vi "Rate scan.vi"(6 "T Ventana":u32 format="%x", 7 "Espera acceso USB":u32, 8 "error in 2":errorcluster, 9 "Valor buscado scalers (5000)":u16, 10 "Sumador":u8, 11 "ftHandle_in 2":u32) -> (0 "error out 2":errorcluster, 1 "DAC\nTH3,TH4,TH5":u16 format="%x", 2 "DAC\nTH0,TH1,TH2":u16 format="%x", 3 "ftHandle_out 2":u32, 5 "Scaler 1":u16)   [LabVIEW 2019]
uses:
  Origen Socket SERVO_PCB_BUENO_v5 (muchos asics)/Global_STOP.vi
panel:
  out "Scaler 2":u16
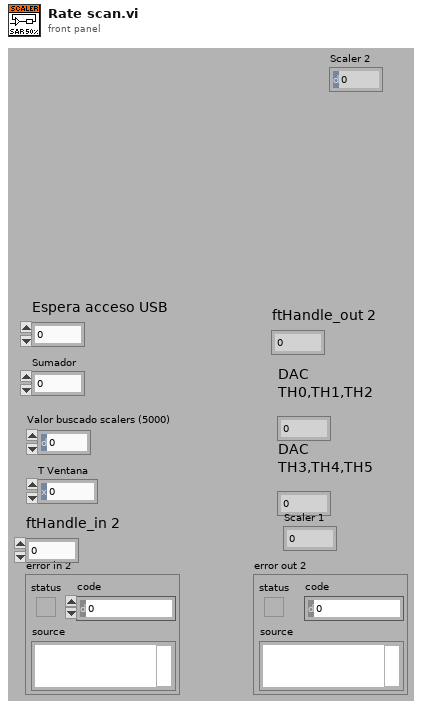
[diagram p1: front panel]
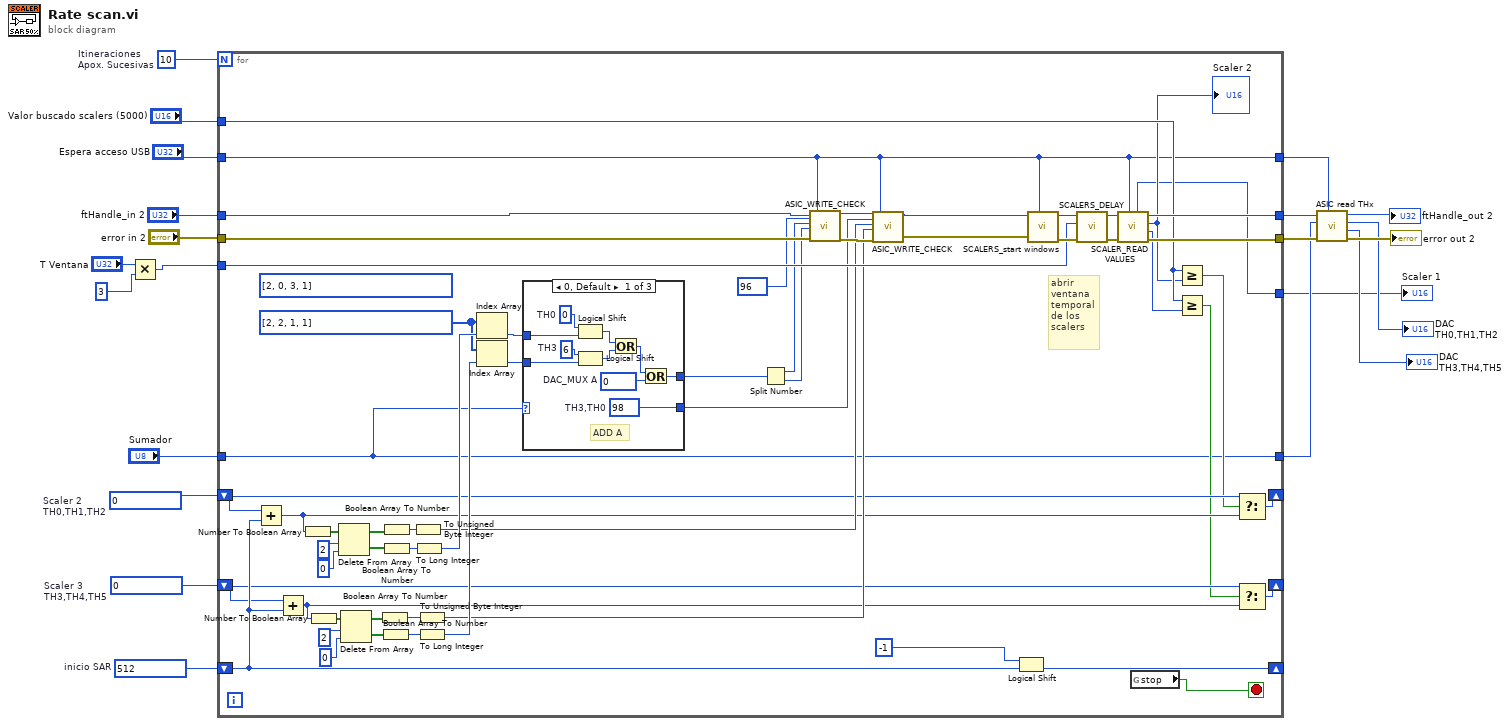
[diagram p0: block diagram]
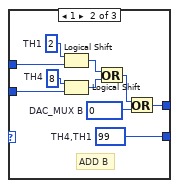
[diagram p2: hidden frame]
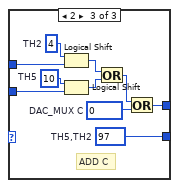
[diagram p3: hidden frame]
diagram:
  w14 = u16 0  # Scaler 3 TH3,TH4,TH5
  w15 = u16 0  # Scaler 2 TH0,TH1,TH2
  w16 = u16 512  # inicio SAR
  w18 = 10  # Itineraciones Apox. Sucesivas
  n1 = Multiply(x="T Ventana", y=u32 3) -> (x*y=w2:u32)
  n2 = for {
    N: w18 -> [_]
    tunnel: "Espera acceso USB" -> [w26]
    tunnel: w2 -> [w76]
    tunnel: "Valor buscado scalers (5000)" -> [w28]
    shift-right: [w72] -> _
    shift-left: w16 -> [w71]
    shift-right: [w33] -> _
    shift-left: w15 -> [w40]
    shift-right: [w32] -> _
    shift-left: w14 -> [w38]
    tunnel: "Sumador" -> [w30]
    tunnel: [w30] -> w9
    tunnel: [w26] -> w10
    tunnel: [w25] -> w4
    tunnel: "ftHandle_in 2" -> [w54]
    tunnel: [w35] -> w11
    tunnel: "error in 2" -> [w53]
    tunnel: [w34] -> w12
    stop <- w22 stop-if-true
    (unwired) u16[] [2, 0, 3, 1]
    w51 = u16[] [2, 2, 1, 1]
    # "abrir ventana temporal de los scalers"
    n3 = Add(x=w40, y=w71) -> (x+y=w39:u16)
    n4 = Add(x=w38, y=w71) -> (x+y=w37:u16)
    n5 = Number To Boolean Array(number=w39) -> (Boolean array=w70:bool[])
    n6 = Number To Boolean Array(number=w37) -> (Boolean array=w69:bool[])
    n7 = Delete From Array(array=w70, length=2, index=0) -> (deleted portion=w63:bool[], array with subset deleted=w68:bool[])
    n8 = Delete From Array(array=w69, length=2, index=0) -> (deleted portion=w61:bool[], array with subset deleted=w62:bool[])
    n9 = Boolean Array To Number(Boolean array=w62) -> (number=w59:u32)
    n10 = Boolean Array To Number(Boolean array=w61) -> (number=w57:u32)
    n11 = Boolean Array To Number(Boolean array=w68) -> (number=w60:u32)
    n12 = Boolean Array To Number(Boolean array=w63) -> (number=w58:u32)
    n13 = To Unsigned Byte Integer(number=w60) -> (unsigned 8bit integer=w42:u8)
    n14 = To Long Integer(number=w58) -> (32bit integer=w56:i32)
    n15 = To Unsigned Byte Integer(number=w59) -> (unsigned 8bit integer=w41:u8)
    n16 = To Long Integer(number=w57) -> (32bit integer=w55:i32)
    n17 = Index Array(array=w51, index=w56) -> (element=w50:u16)
    n18 = Index Array(array=w51, index=w55) -> (element=w49:u16)
    n19 = case shown="0, Default" w30 {
      tunnel: [w88 w98 w108] -> w43
      tunnel: w50 -> [w87 w97 w107]
      tunnel: w49 -> [w86 w96 w106]
      tunnel: [w80 w90 w100] -> w44
      frame 0, Default {
        w79 = u16 0  # DAC_MUX A
        w84 = i8 6  # TH3
        w85 = i8 0  # TH0
        w88 = u8 98  # TH3,TH0
        # "ADD A"
        n20 = Logical Shift(y=w85, x=w87) -> (x << y=w82:u16)
        n21 = Logical Shift(y=w84, x=w86) -> (x << y=w83:u16)
        n22 = Or(x=w82, y=w83) -> (x .or. y?=w81:u16)
        n23 = Or(x=w81, y=w79) -> (x .or. y?=w80:u16)
      }
      frame 1 {
        w89 = u16 0  # DAC_MUX B
        w94 = i8 8  # TH4
        w95 = i8 2  # TH1
        w98 = u8 99  # TH4,TH1
        # "ADD B"
        n24 = Logical Shift(y=w95, x=w97) -> (x << y=w92:u16)
        n25 = Logical Shift(y=w94, x=w96) -> (x << y=w93:u16)
        n26 = Or(x=w92, y=w93) -> (x .or. y?=w91:u16)
        n27 = Or(x=w91, y=w89) -> (x .or. y?=w90:u16)
      }
      frame 2 {
        w99 = u16 0  # DAC_MUX C
        w104 = i8 10  # TH5
        w105 = i8 4  # TH2
        w108 = u8 97  # TH5,TH2
        # "ADD C"
        n28 = Logical Shift(y=w105, x=w107) -> (x << y=w102:u16)
        n29 = Logical Shift(y=w104, x=w106) -> (x << y=w103:u16)
        n30 = Or(x=w102, y=w103) -> (x .or. y?=w101:u16)
        n31 = Or(x=w101, y=w99) -> (x .or. y?=w100:u16)
      }
    }
    n32 = Split Number(x=w44) -> (hi(x)=w45:u8, lo(x)=w46:u8)
    n33 = call "ASIC_WRITE_CHECK.vi"("ftHandle_in"=w54, "Direccion Registro Asic"=u8 96, "Byte Alto"=w45, "Byte Bajo"=w46, "error in"=w53, "Espera acceso USB 2"=w26) -> ("ftHandle_out"=w48:u32, "error out"=w47:errorcluster)  [unwired: 11 in, 1 out]
    n34 = call "ASIC_WRITE_CHECK.vi"("ftHandle_in"=w48, "Direccion Registro Asic"=w43, "Byte Alto"=w42, "Byte Bajo"=w41, "error in"=w47, "Espera acceso USB 2"=w26) -> ("ftHandle_out"=w24:u32, "error out"=w23:errorcluster)  [unwired: 11 in, 1 out]
    n35 = Logical Shift(y=i8 -1, x=w71) -> (x << y=w72:u16)
    n36 = call "SCALERS_start windows.vi"("Espera acceso USB"=w26, "error in 2"=w23, "ftHandle_in 2"=w24) -> ("error out"=w77:errorcluster, "ftHandle_out"=w78:u32)  [unwired: 7 in]
    n37 = call "SCALERS_DELAY.vi"("error out 2"=w77, "Ventana 2"=w76, "ftHandle_out 2"=w78) -> ("error out"=w74:errorcluster, "ftHandle_out"=w75:u32)  [unwired: 7 in]
    n38 = call "SCALER_READ VALUES.vi"("Espera acceso USB"=w26, "error in"=w74, "ftHandle_in"=w75) -> ("error out"=w34:errorcluster, "Scaler 3"=w29:u16, "Scaler 2"=w27:u16, "ftHandle_out"=w35:u32, "Scaler 1"=w25:u16)  [unwired: 3 in, 1 out]
    "Scaler 2" <- w27
    n39 = global read "Global_STOP.vi" "stop"() -> (w22:bool)
    n40 = Greater Or Equal?(x=w28, y=w27) -> (x >= y?=w36:bool)
    n41 = Greater Or Equal?(x=w28, y=w29) -> (x >= y?=w31:bool)
    n42 = Select(t=w40, s=w36, f=w39) -> (s? t:f=w33:u16)
    n43 = Select(t=w38, s=w31, f=w37) -> (s? t:f=w32:u16)
  }
  "Scaler 1" <- w4
  n44 = call "ASIC read THx.vi"("Espera acceso USB"=w10, "error in"=w12, "Sumador"=w9, "ftHandle_in"=w11) -> ("error out 2"=→"error out 2":errorcluster, "THx+3"=→"DAC\nTH3,TH4,TH5":u16, "THx"=→"DAC\nTH0,TH1,TH2":u16, "ftHandle_out 2"=→"ftHandle_out 2":u32)  [unwired: 4 in]
